vi "1-Byte Mono to U8.vi"(0 "1-Byte Mono Data":u8[](array[numeric]) format="%08b", 1 "Image Size":T1) -> (2 "U8 Pixels":u8[][](array[numeric]) format="%08b")   [LabVIEW 2020, in "Buffer.lvclass"]
uses:
  Buffer.lvclass
  Image Size.ctl
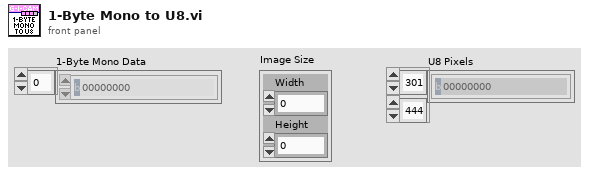
[diagram p1: front panel]
types:
  T1 = typedef "Buffer.lvclass/Image Size.ctl" = cluster{"Width":u16, "Height":u16}
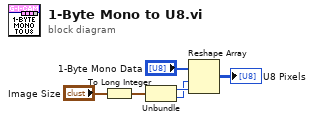
[diagram p0: block diagram]
diagram:
  n1 = To Long Integer(number="Image Size") -> (32bit integer=w2:cluster{"Width":i32, "Height":i32})
  n2 = Unbundle(w2) -> ("Width"=w4:i32, "Height"=w3:i32)
  n3 = Reshape Array("1-Byte Mono Data", w3, w4) -> (→"U8 Pixels":u8[][])
